vi "Reset.vi"(8 "error in (no error)":errorcluster, 10 "Values":refnum<class "Values.lvclass">, 11 "Processing in":refnum<class "Processing.lvclass">) -> (0 "error out":errorcluster, 3 "Processing out":refnum<class "Processing.lvclass">)   [LabVIEW 2020, in "HTTP Server.lvlib" / "Processing.lvclass"]
uses:
  Processing.lvclass
  Processing.lvclass/Processing.ctl
  <vilib>/IlluminatedG/IG HTTP Utils/HTTP Utils/Request/Request.lvclass
  <vilib>/IlluminatedG/IG HTTP Utils/HTTP Utils/Response/Response.lvclass
  RequestTraceLog/RequestTraceLog.lvclass
  Session/Session.lvclass
  HTTP TCP Client/HTTP TCP Client.lvclass
  C:/Program Files (x86)/National Instruments/LabVIEW 2020/vi.lib/IlluminatedG/lv-stream-tcp/TCP Client/TCP Client.lvclass
  C:/Program Files (x86)/National Instruments/LabVIEW 2020/vi.lib/IlluminatedG/lv-stream/Connection/Connection.lvclass
  C:/Program Files (x86)/National Instruments/LabVIEW 2020/vi.lib/IlluminatedG/lv-stream/Endpoint/Endpoint.lvclass
  C:/dev/lv/2020/lv-http-server/HTTP Server/HTTP TCP Client/HTTP TCP Client.lvclass
  Values/Values.lvclass
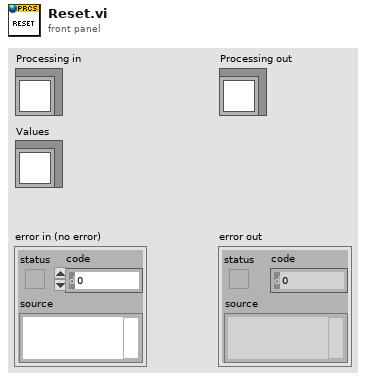
[diagram p1: front panel]
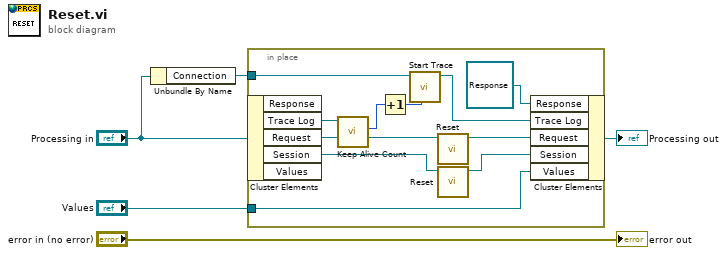
[diagram p0: block diagram]
diagram:
  n1 = Unbundle By Name("Processing in") -> ("Connection"=w2:refnum<class "HTTP TCP Client.lvclass">)
  n2 = in-place {
    in-place-border: w2 -> [w13]
    in-place-border: "Values" -> [w10]
    n3 = in-place-cluster #1("Processing in") -> ("Trace Log"=w9:refnum<class "RequestTraceLog.lvclass">, "Request"=w16:refnum<class "Request.lvclass">, "Session"=w12:refnum<class "Session.lvclass">)  [unwired: 2 out]
    n4 = call "Keep Alive Count.vi"("RequestTraceLog in"=w9) -> ("Keep Alive Count"=w8:i32)  [unwired: 9 in, 1 out]
    n5 = Increment(x=w8) -> (x+1=w6:i32)
    n6 = call "Start Trace.vi"("Keep Alive Count (0)"=w6, "Connection"=w13) -> ("RequestTraceLog out"=w14:refnum<class "RequestTraceLog.lvclass">)  [unwired: 8 in, 1 out]
    n7 = call <vilib>:"Reset.vi"("Request in"=w16) -> ("Request out"=w15:refnum<class "Request.lvclass">)  [unwired: 9 in, 1 out]
    n8 = call <vilib>:"Reset.vi"("Session in"=w12) -> ("Session out"=w11:refnum<class "Session.lvclass">)  [unwired: 9 in, 1 out]
    n9 = in-place-cluster #1("Response"=refnum<class "Response.lvclass"> refnum, "Trace Log"=w14, "Request"=w15, "Session"=w11, "Values"=w10) -> (→"Processing out":refnum<class "Processing.lvclass">)
  }
  "error out" <- "error in (no error)"
